vi "Ramp.vi"(6 "Ramp Interval":dbl, 8 "error in (no error)":errorcluster, 9 "Ramp Duration":dbl, 10 "Ramp End Point":dbl, 11 "PXIe5413 in":refnum<class "PXIe5413.lvclass">) -> (0 "error out":errorcluster, 3 "PXIe5413 out":refnum<class "PXIe5413.lvclass">)   [LabVIEW 2018, in "PXIe5413.lvlib" / "PXIe5413.lvclass"]
uses:
  PXIe5413.lvclass
  PXIe5413.lvclass/PXIe5413.ctl
  <vilib>/Analysis/1siggen.llb/Ramp Pattern by Samples.vi
  <vilib>/Analysis/NI_AALBase.lvlib
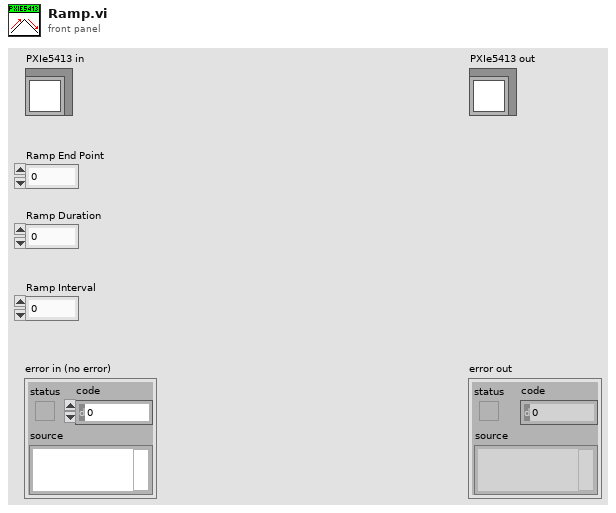
[diagram p1: front panel]
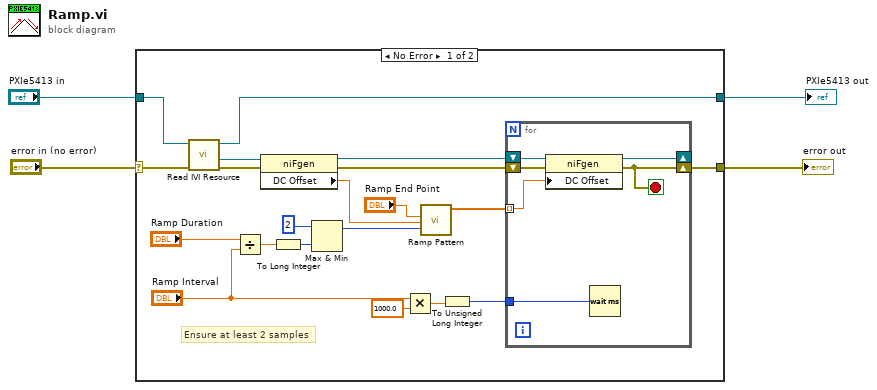
[diagram p0: block diagram]
diagram:
  n1 = case shown="No Error" "error in (no error)" {
    selector: "error in (no error)" -> [w24 w32]
    tunnel: [w7 w32] -> w3
    tunnel: [w6 w31] -> w2
    tunnel: "PXIe5413 in" -> [w23 w31]
    frame No Error {
      # "Ensure at least 2 samples"
      n2 = call "Read IVI Resource.vi"("error in (no error)"=w24, "PXIe5413 in"=w23) -> ("error out"=w21:errorcluster, "IVI Resource"=w22:refnum<k15>, "PXIe5413 out"=w6:refnum<class "PXIe5413.lvclass">)  [unwired: 7 in]
      n3 = Divide(x="Ramp Duration", y="Ramp Interval") -> (x/y=w15:dbl)
      n4 = property class="niFgen"(reference=w22, error in=w21) -> (reference out=w5:refnum<k15>, error out=w8:errorcluster, "DC Offset"=w20:dbl)
      n5 = To Long Integer(number=w15) -> (32bit integer=w16:i32)
      n6 = Max & Min(x=2, y=w16) -> (max(x,y)=w14:i32)  [unwired: 1 out]
      n7 = Multiply(x="Ramp Interval", y=1000.0) -> (x*y=w10:dbl)
      n8 = call-poly <vilib>:"Ramp Pattern.vi"("start"=w20, "end"="Ramp End Point", "samples"=w14) -> ("Ramp Pattern"=w13:dbl[])  [unwired: 7 in, 1 out]
      n9 = To Unsigned Long Integer(number=w10) -> (unsigned 32bit integer=w9:u32)
      n10 = for {
        tunnel: w13 -> [w29] mode=indexing
        tunnel: w9 -> [w30]
        shift-right: [w27] -> w7
        shift-left: w8 -> [w28]
        shift-right: [w25] -> _
        shift-left: w5 -> [w26]
        stop <- w27 stop-if-true
        n11 = property class="niFgen"(reference=w26, error in=w28, "DC Offset"=w29) -> (reference out=w25:refnum<k15>, error out=w27:errorcluster)
        n12 = Wait (ms)(milliseconds to wait=w30) -> ()  [unwired: 1 out]
      }
    }
    frame Error {
    }
  }
  "error out" <- w3
  "PXIe5413 out" <- w2
